vi "GetAttribute.vi"(8 "error in (no error)":errorcluster, 10 "Attribute":string, 11 "ClusterTreeDict in":refnum<class "TreeLUT.lvclass">) -> (0 "error out":errorcluster, 2 "Value":variant, 3 "ClusterTreeDict out":refnum<class "TreeLUT.lvclass">)   [LabVIEW 2017, in "TreeLUT.lvclass"]
uses:
  TreeLUT.lvclass
  TreeLUT.lvclass/TreeLUT.ctl
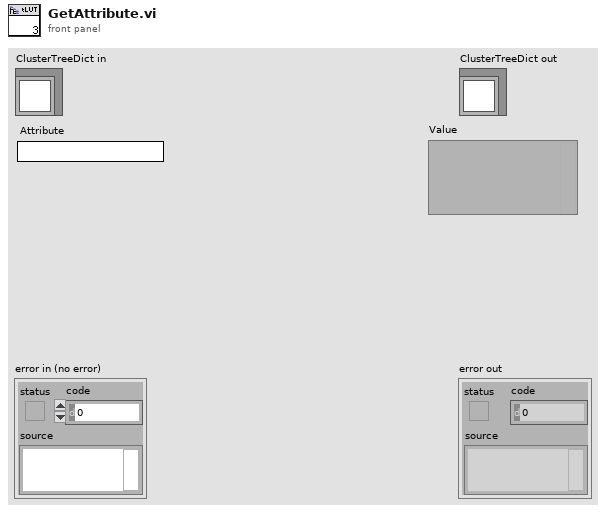
[diagram p1: front panel]
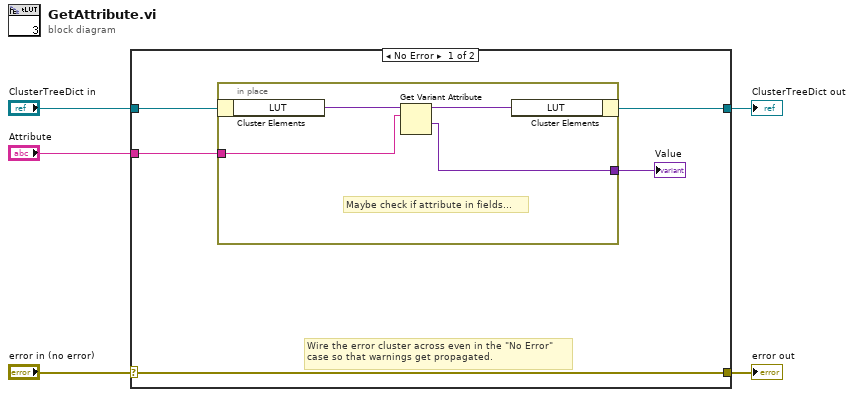
[diagram p0: block diagram]
diagram:
  n1 = case shown="No Error" "error in (no error)" {
    selector: "error in (no error)" -> [w10 w16]
    tunnel: [w10 w16] -> w4
    tunnel: [w6 w15] -> w2
    tunnel: "ClusterTreeDict in" -> [w9 w15]
    tunnel: "Attribute" -> [w8 _]
    frame No Error {
      # "Wire the error cluster across even in the \"No Error\"\ncase so that warnings get propagated."
      n2 = in-place {
        in-place-border: w8 -> [w12]
        in-place-border: [w11] -> w7
        # "Maybe check if attribute in fields..."
        n3 = in-place-cluster #1(w9) -> ("LUT"=w14:variant)
        n4 = Get Variant Attribute(Variant=w14, name=w12) -> (duplicate Variant=w13:variant, value=w11:variant)  [unwired: 2 in, 2 out]
        n5 = in-place-cluster #1("LUT"=w13) -> (w6:refnum<class "TreeLUT.lvclass">)
      }
      "Value" <- w7
    }
    frame Error {
    }
  }
  "error out" <- w4
  "ClusterTreeDict out" <- w2
